vi "Harmonic Analyzer.vi"(4 "fundamental frequency":dbl format="%0.2f", 5 "frame size":i32, 6 "sampling rate":dbl=1.0 format="%0.2f", 7 "window":T1(ring), 8 "# harmonics":i32=5 min=1 step=1, 9 "Auto Power Spectrum":dbl[](array[numeric])) -> (0 "% THD + Noise":dbl format="%0.2f", 1 "% THD":dbl format="%0.2f", 2 "Harmonic Frequencies":dbl[](array[numeric]), 3 "Harmonic Amplitudes":dbl[](array[numeric]))   [LabVIEW 2010, in "NI_AALPro.lvlib"]
doc: "Finds the fundamental and harmonic components (amplitude and frequency) present in the input <B>Auto Power Spectrum</B>, and computes the percent of total harmonic distortion (<B>%THD</B>) and the total harmonic distortion plus noise (<B>%THD + Noise</B>)."
uses:
  NI_AALPro.lvlib
panel:
  # "Harmonic Analyzer"
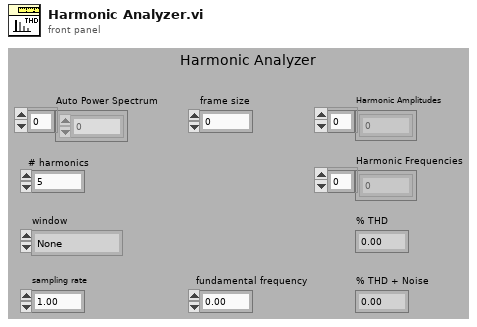
[diagram p1: front panel]
types:
  T1 = enum32{"None ", "Hanning", "Hamming", "Blackman-Harris", "Exact Blackman", "Blackman", "Flat Top", "4 Term B-Harris ", "7 Term B-Harris"}
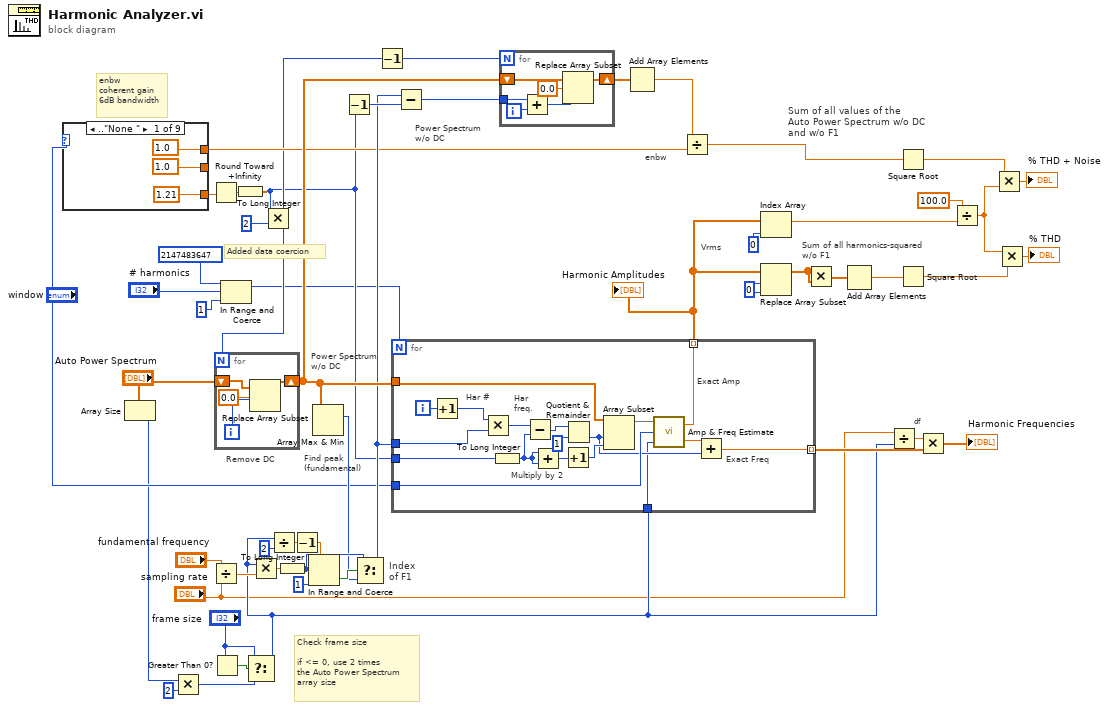
[diagram p0: block diagram]
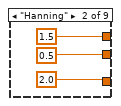
[diagram p2: hidden frame]
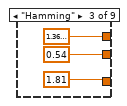
[diagram p3: hidden frame]
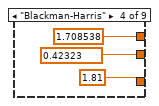
[diagram p4: hidden frame]
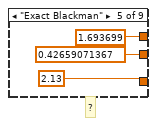
[diagram p5: hidden frame]
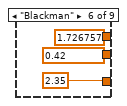
[diagram p6: hidden frame]
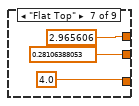
[diagram p7: hidden frame]
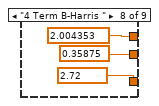
[diagram p8: hidden frame]
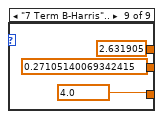
[diagram p9: hidden frame]
diagram:
  w48 = 0
  # "Added data coercion"
  # "Check frame size\n\nif <= 0, use 2 times\nthe Auto Power Spectrum\narray size"
  # "enbw"
  # "enbw\ncoherent gain\n6dB bandwidth"
  # "df"
  # "Sum of all harmonics-squared\nw/o F1"
  # "Vrms"
  # "Sum of all values of the\nAuto Power Spectrum w/o DC\nand w/o F1"
  # "Power Spectrum\nw/o DC"
  # "Index \nof F1"
  # "Power Spectrum\nw/o DC"
  # "Find peak\n(fundamental)"
  # "Remove DC"
  n1 = case shown="..\"None \"" "window" {
    tunnel: [1.0 0.5 0.54 0.42323 0.42659071367 0.42 0.28106388053 0.35875 0.27105140069342415] -> _
    tunnel: [1.0 1.5 1.362826 1.708538 1.693699 1.726757 2.965606 2.004353 2.631905] -> w16
    tunnel: [1.21 2.0 1.81 1.81 2.13 2.35 4.0 2.72 4.0] -> w15
    frame .."None " {
    }
    frame "Hanning" {
    }
    frame "Hamming" {
    }
    frame "Blackman-Harris" {
    }
    frame "Exact Blackman" {
      # "?"
    }
    frame "Blackman" {
    }
    frame "Flat Top" {
      # "?"
    }
    frame "4 Term B-Harris " {
    }
    frame "7 Term B-Harris".. {
      # "?"
    }
  }
  n2 = Array Size(array="Auto Power Spectrum") -> (size(s)=w10:i32)
  n3 = Multiply(x=w10, y=2) -> (x*y=w8:i32)
  n4 = Round Toward +Infinity(x=w15) -> (ceil(x): smallest int >= x=w12:dbl)
  n5 = Divide(x="fundamental frequency", y="sampling rate") -> (x/y=w22:dbl)
  n6 = Greater Than 0?(x="frame size") -> (x > 0?=w11:bool)
  n7 = In Range and Coerce(upper limit=2147483647, x="# harmonics", lower limit=1) -> (coerced(x)=w2:i32)  [unwired: 1 out]
  n8 = To Long Integer(number=w12) -> (32bit integer=w5:i32)
  n9 = Select(t="frame size", s=w11, f=w8) -> (s? t:f=w6:i32)
  n10 = Multiply(x=w6, y=w22) -> (x*y=w32:dbl)
  n11 = Multiply(x=w5, y=2) -> (x*y=w13:i32)
  n12 = for {
    N: w13 -> [_]
    shift-right: [w82] -> w40
    shift-left: "Auto Power Spectrum" -> [w81]
    i -> [w84]
    n13 = Replace Array Subset(array=w81, new element=0.0, index=w84) -> (w82:dbl[])
  }
  n14 = Divide(x=w6, y=2) -> (x/y=w34:dbl)
  n15 = To Long Integer(number=w32) -> (32bit integer=w30:i32)
  n16 = Decrement(x=w34) -> (x-1=w33:dbl)
  n17 = In Range and Coerce(upper limit=w33, x=w30, lower limit=1) -> (In Range?=w31:bool)  [unwired: 1 out]
  n18 = Array Max & Min(array=w40) -> (max index (indices)=w28:i32)  [unwired: 3 out]
  n19 = Decrement(x=w5) -> (x-1=w41:i32)
  n20 = Select(t=w30, s=w31, f=w28) -> (s? t:f=w29:i32)
  n21 = Decrement(x=w13) -> (x-1=w42:i32)
  n22 = for {
    N: w2 -> [_]
    tunnel: w40 -> [w98]
    tunnel: "window" -> [w96]
    tunnel: [w94] -> w23 mode=indexing
    tunnel: [w93] -> w25 mode=indexing
    tunnel: w29 -> [w87]
    tunnel: w6 -> [w86]
    tunnel: w5 -> [w85]
    i -> [w95]
    # "Multiply by 2"
    # "Exact Amp"
    # "Exact Freq"
    # "Har\nfreq."
    # "Har #"
    n23 = Increment(x=w95) -> (x+1=w88:i32)
    n24 = Multiply(x=w88, y=w87) -> (x*y=w102:i32)
    n25 = To Long Integer(number=w85) -> (32bit integer=w101:i32)
    n26 = Subtract(x=w102, y=w101) -> (x-y=w90:i32)
    n27 = Add(x=w101, y=w101) -> (x+y=w100:i32)
    n28 = Increment(x=w100) -> (x+1=w99:i32)
    n29 = Quotient & Remainder(x=w90, y=1) -> (floor(x/y)=w91:i32)  [unwired: 1 out]
    n30 = Array Subset(array=w98, index=w91, length=w99) -> (w97:dbl[])
    n31 = call "Amp & Freq Estimate.vi"("Size of FFT"=w86, "window"=w96, "Part of Power Spectrum"=w97) -> ("Exact Freq Index"=w92:dbl, "Exact Amplitude (Vrms)"=w94:dbl)
    n32 = Add(x=w92, y=w91) -> (x+y=w93:dbl)
  }
  "Harmonic Amplitudes" <- w23
  n33 = Subtract(x=w29, y=w41) -> (x-y=w37:i32)
  n34 = for {
    N: w42 -> [_]
    shift-right: [w107] -> w39
    shift-left: w40 -> [w106]
    tunnel: w37 -> [w103]
    i -> [w105]
    n35 = Add(x=w103, y=w105) -> (x+y=w104:i32)
    n36 = Replace Array Subset(array=w106, new element=0.0, index=w104) -> (w107:dbl[])
  }
  n37 = Add Array Elements(numeric array=w39) -> (sum=w45:dbl)
  n38 = Divide(x=w45, y=w16) -> (x/y=w38:dbl)
  n39 = Index Array(array=w23, index=0) -> (element=w20:dbl)
  n40 = Replace Array Subset(array=w23, new element=w48, index=w48) -> (w47:dbl[])
  n41 = Multiply(x=w47, y=w47) -> (x*y=w51:dbl[])
  n42 = Add Array Elements(numeric array=w51) -> (sum=w50:dbl)
  n43 = Divide(x="sampling rate", y=w6) -> (x/y=w26:dbl)
  n44 = Square Root(x=w38) -> (sqrt(x)=w43:dbl)
  n45 = Square Root(x=w50) -> (sqrt(x)=w18:dbl)
  n46 = Multiply(x=w26, y=w25) -> (x*y=→"Harmonic Frequencies":dbl[])
  n47 = Divide(x=100.0, y=w20) -> (x/y=w19:dbl)
  n48 = Multiply(x=w43, y=w19) -> (x*y=→"% THD + Noise":dbl)
  n49 = Multiply(x=w19, y=w18) -> (x*y=→"% THD":dbl)
